vi "ItemClickedCallback.vi"(4 "MenuStrip out":refnum<class "MGI_MenuStrip.lvclass">, 5 "Event Data":cluster{"sender":refnum<k24>, "e":refnum<k24>}, 6 "Control Ref":refnum<k24>, 7 "Event Common Data":T1) -> ()   [LabVIEW 2016, in "MGI_MenuStrip.lvclass"]
doc: "Authored by Derek E. Trepanier\nsupport@mooregoodideas.com\nwww.mooregoodideas.com\n\nCopyright (c) 2012, Moore Good Ideas, Inc.\n\nAll rights reserved.\n\nRedistribution and use in source and binary forms, with or without modification, are permitted provided that the following conditions are met:\n\n * Redistributions of source code must retain the above copyright notice, this list of conditions and the following disclaimer.\n * Redistributions in binary form must reproduce the above copyright notice, this list of conditions and the following disclaimer in the documentation and/or other materials provided with the distribution.\n * Neither the name of Moore Good Ideas, Inc. nor the names of its contributors may be used to endorse or promote products derived from this software without specific prior written permission.\n\nTHIS SOFTWARE IS PROVIDED BY THE COPYRIGHT HOLDERS AND CONTRIBUTORS \"AS IS\" AND ANY EXPRESS OR IMPLIED WARRANTIES, INCLUDING, BUT NOT LIMITED TO, THE IMPLIED WARRANTIES OF MERCHANTABILITY AND FITNESS FOR A PARTICULAR PURPOSE ARE DISCLAIMED. IN NO EVENT SHALL THE COPYRIGHT OWNER OR CONTRIBUTORS BE LIABLE FOR ANY DIRECT, INDIRECT, INCIDENTAL, SPECIAL, EXEMPLARY, OR CONSEQUENTIAL DAMAGES (INCLUDING, BUT NOT LIMITED TO, PROCUREMENT OF SUBSTITUTE GOODS OR SERVICES; LOSS OF USE, DATA, OR PROFITS; OR BUSINESS INTERRUPTION) HOWEVER CAUSED AND ON ANY THEORY OF LIABILITY, WHETHER IN CONTRACT, STRICT LIABILITY, OR TORT (INCLUDING NEGLIGENCE OR OTHERWISE) ARISING IN ANY WAY OUT OF THE USE OF THIS SOFTWARE, EVEN IF ADVISED OF THE POSSIBILITY OF SUCH DAMAGE."
uses:
  <userlib>/_MGI/Menu Building/MenuTypes/MenuStrip/MGI_MenuStrip.lvclass
  System.Windows.Forms
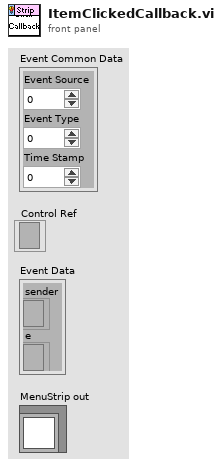
[diagram p1: front panel]
types:
  T1 = cluster{"Event Source":i32, "Event Type":u32, "Time Stamp":u32}
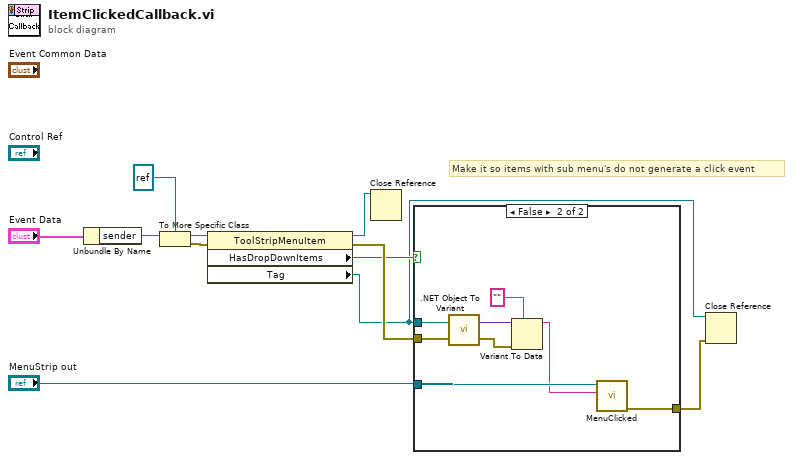
[diagram p0: block diagram]
diagram:
  # "Make it so items with sub menu's do not generate a click event"
  n1 = Unbundle By Name("Event Data") -> ("sender"=w10:refnum<k24>)
  n2 = To More Specific Class(target class=refnum<k24> refnum ("new reference"), reference=w10) -> (specific class reference=w9:refnum<k24>, error out=w8:errorcluster)  [unwired: 1 in]
  n3 = property class="ToolStripMenuItem"(reference=w9, error in=w8) -> (reference out=w1:refnum<k24>, error out=w5:errorcluster, "HasDropDownItems"=w4:bool, "Tag"=w3:refnum<k24>)
  n4 = Close Reference(reference=w1) -> ()  [unwired: 1 in, 1 out]
  n5 = case shown="False" w4 {
    tunnel: "MenuStrip out" -> [_ w19]
    tunnel: w3 -> [_ w18]
    tunnel: w5 -> [_ w17]
    tunnel: [_ w12] -> w2
    frame True {
    }
    frame False {
      n6 = call <vilib>:".NET Object To Variant.vi"("error in (no error)"=w17, ".NET object"=w18) -> ("error out"=w15:errorcluster, "variant"=w16:variant)
      n7 = Variant To Data(error in=w15, type="", Variant=w16) -> (data=w13:string)  [unwired: 1 out]
      n8 = call-dynamic "MenuClicked.vi"("Full Tag"=w13, "Menu in"=w19) -> ("error out"=w12:errorcluster)  [unwired: 8 in, 1 out]
    }
  }
  n9 = Close Reference(reference=w3, error in (no error)=w2) -> ()  [unwired: 1 out]
